vi "6-s.vi"() -> ()   [LabVIEW 2017]
panel:
  out "波形图表":dbl(graph)
  in  "停止":bool
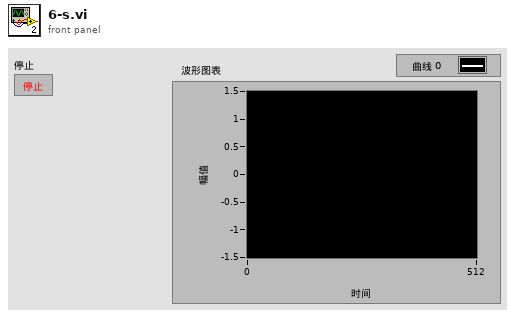
[diagram p1: front panel]
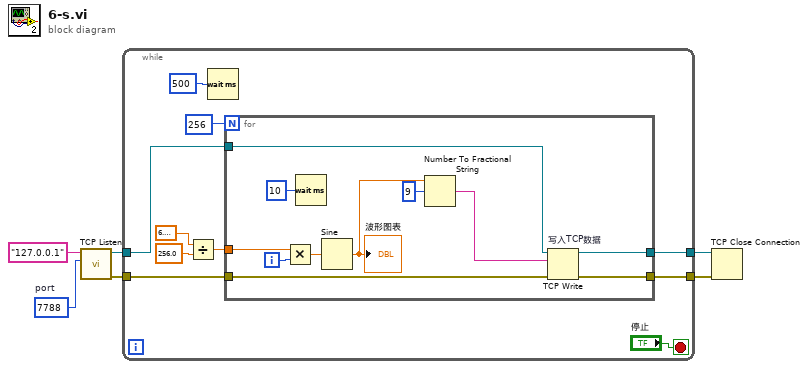
[diagram p0: block diagram]
diagram:
  w6 = u16 7788  # port
  n1 = call <vilib>:"TCP Listen.vi"("port"=w6, "service name"="127.0.0.1") -> ("error out"=w4:errorcluster, "connection ID"=w3:refnum<k5>)  [unwired: 5 in, 3 out]
  n2 = while {
    tunnel: w4 -> [w10]
    tunnel: w3 -> [w9]
    tunnel: [w8] -> w2
    tunnel: [w7] -> w1
    stop <- "停止" stop-if-true
    n3 = Divide(x=6.283185307179586, y=256.0) -> (x/y=w11:dbl)
    n4 = Wait (ms)(milliseconds to wait=u32 500 ("等待时间（毫秒）")) -> ()  [unwired: 1 out]
    n5 = for {
      N: 256 -> [_]
      tunnel: w11 -> [w27]
      tunnel: w10 -> [w24]
      tunnel: w9 -> [w23]
      tunnel: [w22] -> w8
      tunnel: [w21] -> w7
      i -> [w26]
      n6 = Multiply(x=w27, y=w26) -> (x*y=w25:dbl)
      n7 = Wait (ms)(milliseconds to wait=u32 10 ("等待时间（毫秒）")) -> ()  [unwired: 1 out]
      n8 = Sine(x=w25) -> (sin(x)=w20:dbl)
      "波形图表" <- w20
      n9 = Number To Fractional String(number=w20, width (-)=i16 9 ("宽度(-)")) -> (F-format string=w17:string)  [unwired: 2 in]
      n10 = TCP Write "写入TCP数据"(connection ID=w23, data in=w17, error in (no error)=w24) -> (connection ID out=w21:refnum<k5>, error out=w22:errorcluster)  [unwired: 1 in, 1 out]
    }
  }
  n11 = TCP Close Connection(connection ID=w1, error in (no error)=w2) -> ()  [unwired: 1 in, 2 out]
